vi "Eval_MuliVar.vi"(8 "error in (no error)":errorcluster, 9 "varValues":dbl[](array[numeric]) format="%#_13g", 10 "varNames":string[](array[string]), 11 "muExpr in":refnum<class "mupExpr.lvclass">) -> (0 "error out":errorcluster, 2 "Result":dbl format="%#_13g", 3 "muExpr out":refnum<class "mupExpr.lvclass">)   [LabVIEW 2015, in "mupExpr.lvclass"]
uses:
  mupExpr.lvclass
  mupExpr.lvclass/mupExpr.ctl
  Set Variable Value.vi
  mupLib/mupEval.vi
  mupLib/mupSetVarValue.vi
  mupLib/mupCheckError.vi
  mupLib/mupLibPath.vi
  <vilib>/Utility/error.llb/Error Cluster From Error Code.vi
panel:
  # "Update the value of multiple variables then evaluate the expression"
  # "If the variables are not found in the expression, an error will be generated"
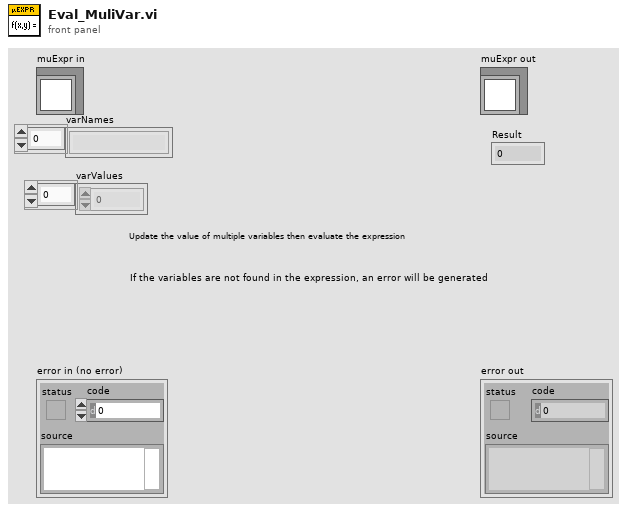
[diagram p1: front panel]
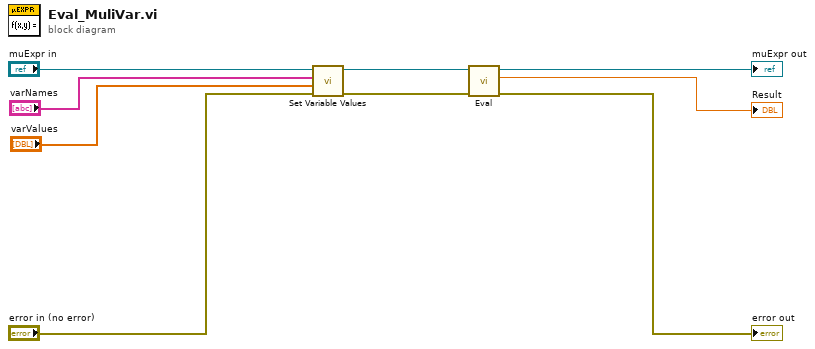
[diagram p0: block diagram]
diagram:
  n1 = call "Set Variable Values.vi"("error in (no error)"="error in (no error)", "varValues"="varValues", "varNames"="varNames", "muExpr in"="muExpr in") -> ("error out"=w2:errorcluster, "muExpr out"=w3:refnum<class "mupExpr.lvclass">)  [unwired: 6 in]
  n2 = call "Eval.vi"("error in (no error)"=w2, "muExpr in"=w3) -> ("error out"=→"error out":errorcluster, "Result"=→"Result":dbl, "muExpr out"=→"muExpr out":refnum<class "mupExpr.lvclass">)  [unwired: 7 in]
